vi "PID Multi-Channel PID Frame 1.vi"(0 "ie(k-1)":i32, 1 "integral gain (Kc*Ts/Ti) (k)":i16, 5 "[e(k)+e(k-1)]/2":i16) -> (4 "u_i(k)":i32, 10 "integration off":bool)   [LabVIEW 2017, in "NI_PID_FPGA.lvlib"]
uses:
  <vilib>/addons/control/pid/NI_PID_FPGA.lvlib
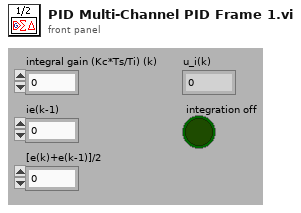
[diagram p1: front panel]
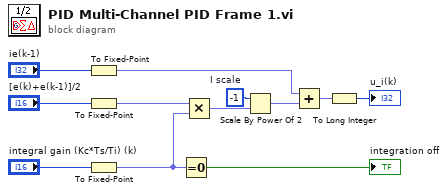
[diagram p0: block diagram]
diagram:
  w1 = i8 -1  # I scale
  n1 = To Fixed-Point(number="ie(k-1)") -> (fixed-point=w6:fxp<+/-,32,32>)  [unwired: 1 in]
  n2 = To Fixed-Point(number="[e(k)+e(k-1)]/2") -> (fixed-point=w8:fxp<+/-,16,16>)  [unwired: 1 in]
  n3 = To Fixed-Point(number="integral gain (Kc*Ts/Ti) (k)") -> (fixed-point=w7:fxp<+/-,16,16>)  [unwired: 1 in]
  n4 = Equal To 0?(x=w7) -> (x = 0?=→"integration off":bool)
  n5 = Multiply(x=w8, y=w7) -> (x*y=w9:fxp<+/-,32,32>)
  n6 = Scale By Power Of 2(n=w1, x=w9) -> (x*2^n=w11:fxp<+/-,32,32>)
  n7 = Add(x=w6, y=w11) -> (x+y=w10:fxp<+/-,32,32>)
  n8 = To Long Integer(number=w10) -> (32bit integer=→"u_i(k)":i32)
